vi "G#Object_GetClassHierarchy.vi"(0 "reference in":refnum<class "G#Object.lvclass">, 5 "error in (no error)":errorcluster) -> (14 "reference out":refnum<class "G#Object.lvclass">, 15 "class hierarchy":T1[](array[typedef]), 19 "error out":errorcluster)   [LabVIEW 2020, in "G#Object.lvclass"]
doc: "Returns the class hierarchy of the given object reference."
uses:
  G#Object.lvclass
  G#Object_ClassHierarchy.ctl
  G#Object_State.ctl
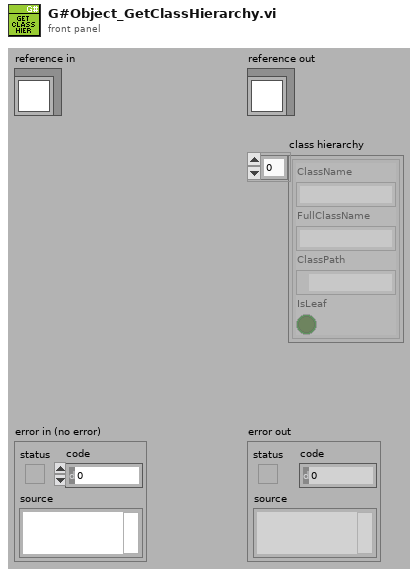
[diagram p1: front panel]
types:
  T1 = typedef "G#Object.lvclass/G#Object_ClassHierarchy.ctl" = cluster{"ClassName":string, "FullClassName":string, "ClassPath":path, "IsLeaf":bool}
  T2 = typedef "G#Object.lvclass/G#Object_State.ctl" = enum16{"Clear", "Create", "Delete", "Get class attributes", "Class hierarchy", "Get attribute value", "Set attribute value"}
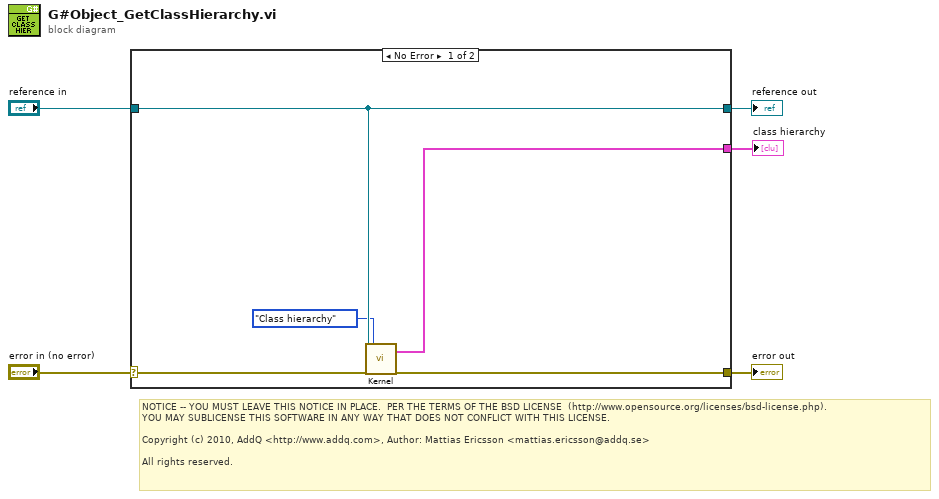
[diagram p0: block diagram]
diagram:
  # "NOTICE -- YOU MUST LEAVE THIS NOTICE IN PLACE.  PER THE TERMS OF THE BSD LICENSE  (http://www.opensource.org/licenses/bsd-license.php).\nYOU MAY SUBLICENSE THIS SOFTWARE IN ANY WAY THAT DOES NOT CONFLICT WITH THIS LICENSE.\n\nCopyright (c) 2010, AddQ <http://www.addq.com>, Author: Mattias Ericsson <mattias.ericsson@addq.se>\n\nAll rights reserved."
  n1 = case shown="No Error" "error in (no error)" {
    selector: "error in (no error)" -> [w10 w12]
    tunnel: [w9 w12] -> w4
    tunnel: [w8 w11] -> w2
    tunnel: "reference in" -> [w8 w11]
    tunnel: [w6 _] -> w1
    frame No Error {
      n2 = call-dynamic "Kernel.vi"("reference in"=w8, "error in (no error)"=w10, "state"=G#Object_State."Class hierarchy" ("State")) -> ("class hierarchy"=w6:T1[], "error out"=w9:errorcluster)  [unwired: 8 in, 7 out]
    }
    frame Error {
    }
  }
  "error out" <- w4
  "reference out" <- w2
  "class hierarchy" <- w1
